vi "Prober_ChuckStatusCheck.vi"(8 "error in (no error)":errorcluster, 11 "SemiProbe in":refnum<class "SemiProbe.lvclass">) -> (0 "error out":errorcluster, 2 "Chuck at CONTACT?":bool=TRUE, 3 "SemiProbe out":refnum<class "SemiProbe.lvclass">)   [LabVIEW 2018, in "SemiProbe.lvclass"]
uses:
  SemiProbe.lvclass
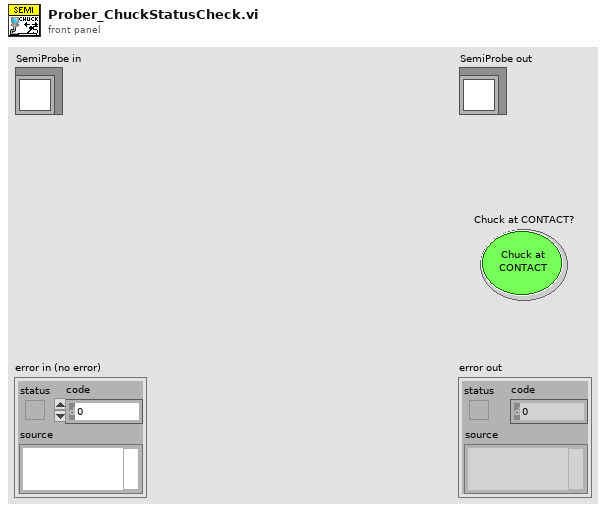
[diagram p1: front panel]
types:
  T1 = cluster{"SP Load Less Than Thr?":bool, "SP Load Threshold (um)":dbl, "SP Current Location":cluster{"X (um)":ext, "Y (um)":ext, "Z (um)":ext, "T (degree)":ext}, "SP Chuck Speeds":cluster{"XY Speed (10-100%)":dbl, "Z Speed (10-100%)":dbl, "T Speed (10-100%)":dbl}, "Manual Step Parameters":cluster{"Step in X":bool, "X S-Speed [µm/step]":sgl, "Step in Y":bool, "Y S-Speed [µm/step]":sgl, "Step in Z":bool, "Z S-Speed [µm/step]":sgl, "Step in T":bool, "T S-Speed [mdegree/step]":sgl, "X Increase":bool, "Y Increase?":bool, "Z Increase?":bool, "T Increase?":bool}, "Z Stepper":cluster{"UP/DOWN":bool, "UP/DOWN Speed [µm/step]":i32, "SP Z Step":bool}, "Z Heights Set":bool, "SP Contact Search":cluster{"Contact Circuit":enum16{"12", "1", "2"}, "Speed [1000-10000]":sgl, "Start Height [µm]":sgl, "Search Band [µm]":sgl, "Overdrive [µm]":sgl}, "Separation Distance [µm]":u32, "Contact Height [µm]":u32, "Use Overdrive?":bool, "Touchdown method":enum16{"no feedback", "Arduino edgesense", "SP contact circuit"}, "Arduino Edgesense params":cluster{"touchdown height [µm]":i32, "search band [µm]":u32, "speed [µm/step]":u32, "overdrive [µm]":u32}}
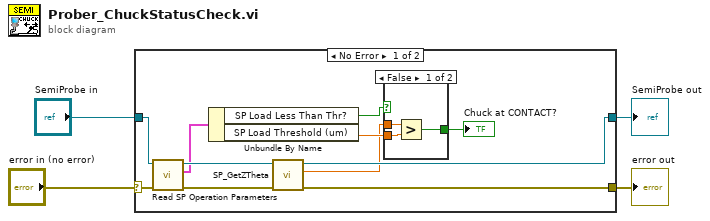
[diagram p0: block diagram]
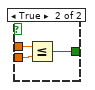
[diagram p2: hidden frame]
diagram:
  n1 = case shown="No Error" "error in (no error)" {
    selector: "error in (no error)" -> [w12 w23]
    tunnel: "SemiProbe in" -> [w13 w22]
    tunnel: [w9 w22] -> w2
    tunnel: [w10 w23] -> w1
    frame No Error {
      n2 = call-dynamic "Read SP Operation Parameters.vi"("error in (no error)"=w12, "SemiProbe in"=w13) -> ("error out"=w15:errorcluster, "SP Operation Parameters"=w11:T1, "SemiProbe out"=w14:refnum<class "SemiProbe.lvclass">)  [unwired: 7 in]
      n3 = Unbundle By Name(w11) -> ("SP Load Less Than Thr?"=w8:bool, "SP Load Threshold (um)"=w7:dbl)
      n4 = call-dynamic "SP_GetZTheta.vi"("error in (no error)"=w15, "SemiProbe in"=w14) -> ("error out"=w10:errorcluster, "Z out [µm]"=w6:dbl, "SemiProbe out"=w9:refnum<class "SemiProbe.lvclass">)  [unwired: 6 in, 1 out]
      n5 = case shown="False" w8 {
        tunnel: w7 -> [w17 w21]
        tunnel: w6 -> [w18 w20]
        tunnel: [w16 w19] -> w5
        frame False {
          n6 = Greater?(x=w18, y=w17) -> (0:w16:bool)
        }
        frame True {
          n7 = Less Or Equal?(x=w20, y=w21) -> (x <= y?=w19:bool)
        }
      }
      "Chuck at CONTACT?" <- w5
    }
    frame Error {
    }
  }
  "error out" <- w1
  "SemiProbe out" <- w2
